vi "Write Topologies.vi"(10 "Topologies in":T1[](array[typedef]), 11 "SLSC Switch in":refnum<class "SLSC Switch.lvclass">) -> (3 "SLSC Switch out":refnum<class "SLSC Switch.lvclass">)   [LabVIEW 2015, in "SLSC Switch.lvlib" / "SLSC Switch.lvclass"]
uses:
  SLSC Switch.lvclass
  Controls/JSON.InitialState.ctl
  Controls/Topology.ctl
  Controls/JSON.ChannelList.ctl
  Controls/JSON.ConnectionList.ctl
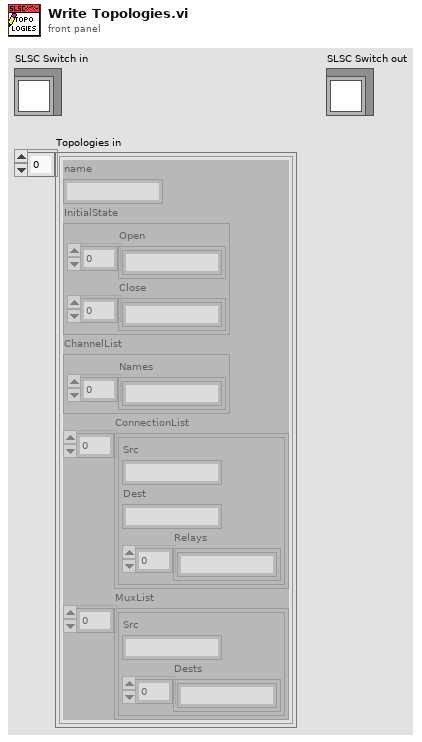
[diagram p1: front panel]
types:
  T1 = typedef "SLSC Switch.lvlib/SLSC Switch.lvclass/Topology.ctl" = cluster{"name":string, "InitialState":T2, "ChannelList":T3, "ConnectionList":T4[], "MuxList":cluster{"Src":string, "Dests":string[]}[]}
  T2 = typedef "SLSC Switch.lvlib/SLSC Switch.lvclass/JSON.InitialState.ctl" = cluster{"Open":string[], "Close":string[]}
  T3 = typedef "SLSC Switch.lvlib/SLSC Switch.lvclass/JSON.ChannelList.ctl" = cluster{"Names":string[]}
  T4 = typedef "SLSC Switch.lvlib/SLSC Switch.lvclass/JSON.ConnectionList.ctl" = cluster{"Src":string, "Dest":string, "Relays":string[]}
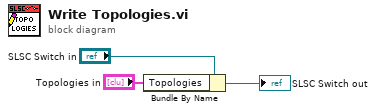
[diagram p0: block diagram]
diagram:
  n1 = Bundle By Name(cluster="SLSC Switch in", "Topologies"="Topologies in") -> (→"SLSC Switch out":refnum<class "SLSC Switch.lvclass">)
